vi "DoInit.vi"(8 "error in (no error)":errorcluster, 11 "Snake in":refnum<class "SnakeGame.lvclass">) -> (0 "error out":errorcluster, 3 "Snake out":refnum<class "SnakeGame.lvclass">)   [LabVIEW 2019, in "RT_Game.lvlib" / "SnakeGame.lvclass"]
uses:
  SnakeGame.lvclass
  C:/Users/FreshBob/Dropbox/VIs/myRIO_GameConsole/RT/RT_Game/Game/Game.lvclass
  SnakeData.ctl
  Direction.ctl
  Game/Coordinate.ctl
  CoordinateData.ctl
  RT_Sprite/RT_Sprite.lvclass
  C:/Users/FreshBob/Dropbox/VIs/myRIO_GameConsole/RT/RT_Game/GameObject/GameObject.lvclass
  PongSwitch/SnakeSwitch.lvclass
  Snake/Snake.lvclass
  SnakeGame.lvclass/SnakeGame.ctl
  GameObject/GameObject.lvclass/GameObject.ctl
  PongSwitch/SnakeSwitch.lvclass/SnakeSwitch.ctl
  Snake/Snake.lvclass/Snake.ctl
  Game/Game.lvclass/Game.ctl
  Snake/Write Position (Tiles).vi
  Snake/Write Direction.vi
  Snake/Write ScorePosition.vi
  Snake/Write Color.vi
  Snake/Write Length.vi
  GameObject/Write name.vi
  PongSwitch/Write Static.vi
  GameObject/Write IsActive.vi
  PongSwitch/Write DisabledTime.vi
  PongSwitch/Write EnabledTime.vi
  PongSwitch/Write randomness.vi
  GameObject/Write Collides_.vi
  Snake/Write Dead_.vi
  GameObject/Read position.vi
  Game/Write Sprites.vi
  Game/Game.lvclass
  GameObject/GameObject.lvclass
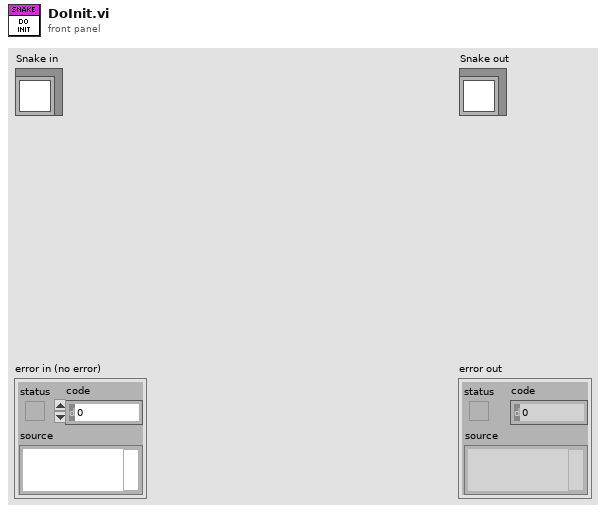
[diagram p1: front panel]
types:
  T1 = typedef "RT_Game.lvlib/Game.lvclass/Coordinate.ctl" = cluster{"x":dbl, "y":dbl}
  T2 = typedef "RT_Game.lvlib/SnakeGame.lvclass/Direction.ctl" = enum16{"Up", "Left", "Down", "Right"}
  T3 = typedef "RT_Game.lvlib/SnakeGame.lvclass/SnakeData.ctl" = cluster{"Length":i16, "Direction":T2, "Position":T1, "Coordinates":T4[], "ScorePosition":T1, "Dead?":bool, "Color":fxp<+,3,3>, "LastDirection":T2}
  T4 = typedef "RT_Game.lvlib/SnakeGame.lvclass/CoordinateData.ctl" = cluster{"Coordinate":T1, "TileCode":u16}
  T5 = cluster{"GameObject out":refnum<class "RT_Sprite.lvclass">, "GameObject out":refnum<class "RT_Sprite.lvclass">, "GameObject out":refnum<class "RT_Sprite.lvclass">}
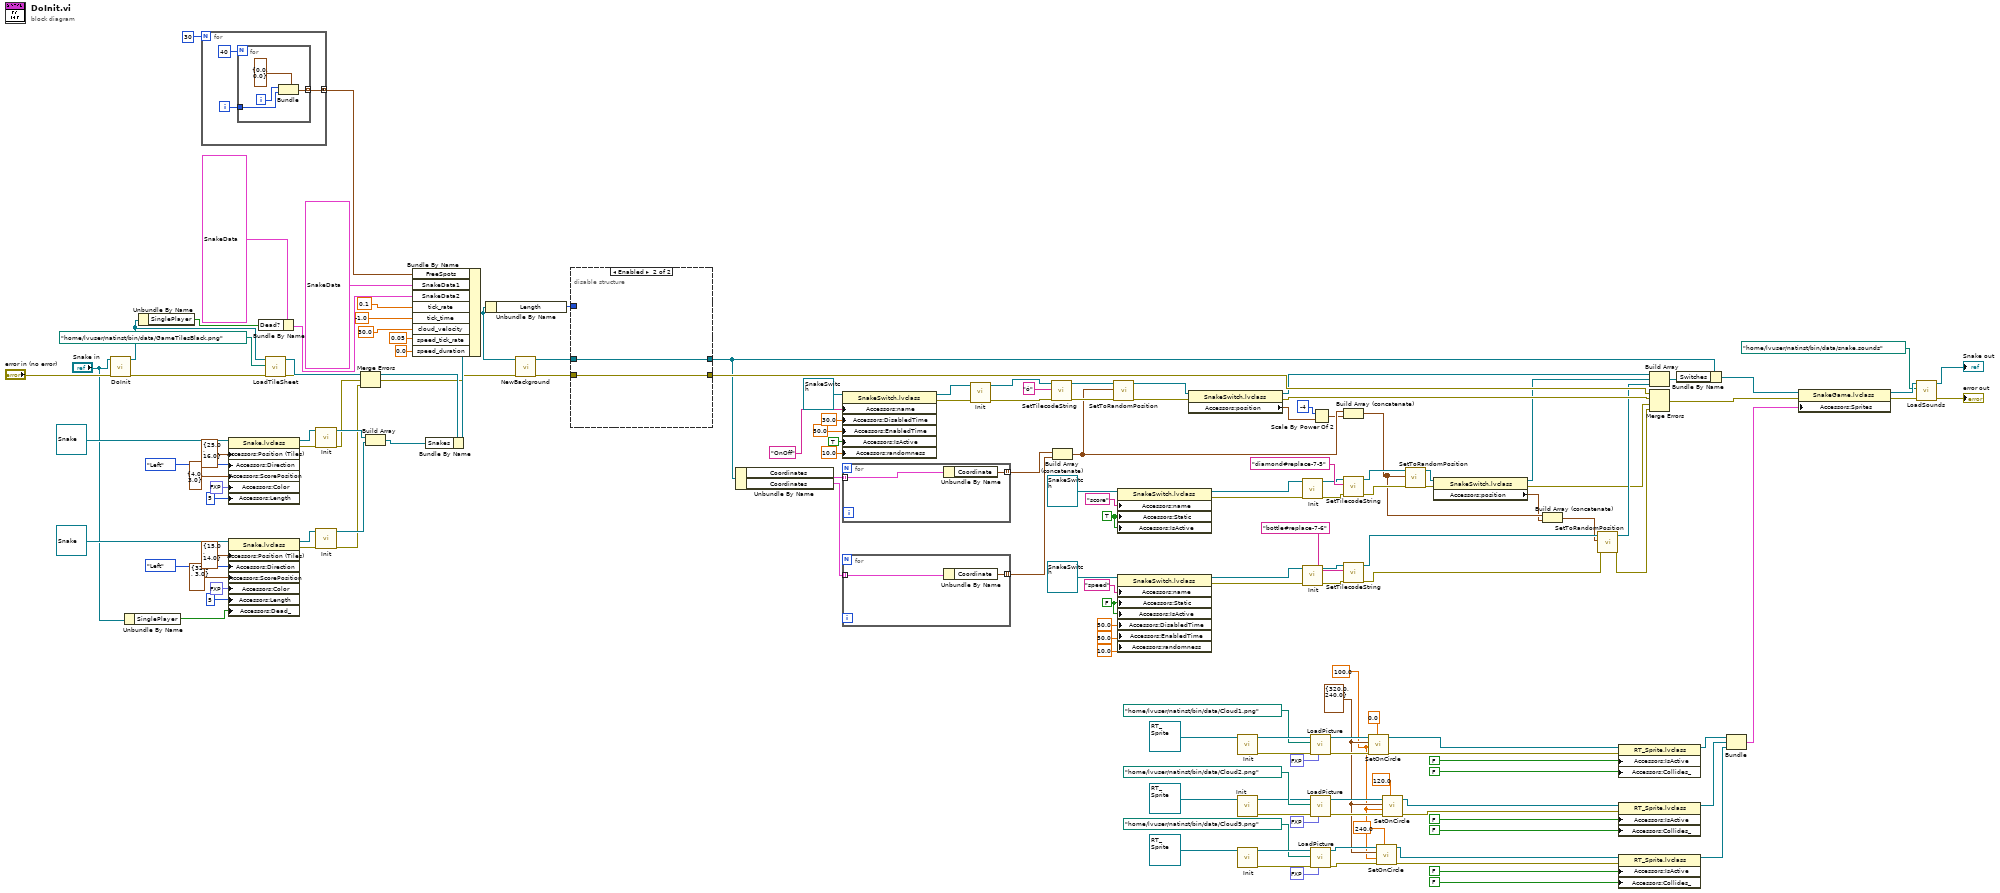
[diagram p0: block diagram]
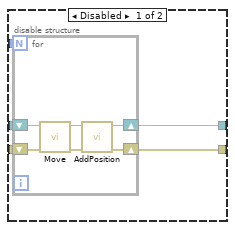
[diagram p2: hidden frame]
diagram:
  w52 = FALSE ("Static")
  w34 = TRUE ("Static")
  w65 = 100.0 ("Radius")
  w66 = T1 {"x"=320.0, "y"=240.0} ("Center")
  n1 = call-parent "DoInit.vi"("error in (no error)"="error in (no error)", "Game in"="Snake in") -> ("error out"=w153:errorcluster, "Game out"=w58:refnum<class "SnakeGame.lvclass">)  [unwired: 8 in]
  n2 = Unbundle By Name("Snake in") -> ("SinglePlayer"=w1:bool)
  n3 = Unbundle By Name(w58) -> ("SinglePlayer"=w146:bool)
  n4 = for {
    N: 30 -> [_]
    tunnel: [w156] -> w28 mode=concatenating
    i -> [w157]
    n5 = for {
      N: 40 -> [_]
      tunnel: w157 -> [w160]
      tunnel: [w159] -> w156 mode=indexing
      i -> [w161]
      n6 = Bundle(cluster=T1 {"x"=0.0, "y"=0.0} ("Coordinate"), "x"=w161, "y"=w160) -> (w159:T1)
    }
  }
  n7 = property class="Snake.lvclass"(reference=refnum<class "Snake.lvclass"> refnum ("RT_Game.lvlib:Snake.lvclass"), "Accessors:Position (Tiles)"=T1 {"x"=25.0, "y"=16.0} ("Position (Tiles)"), "Accessors:Direction"=Direction."Left" ("Direction"), "Accessors:ScorePosition"=T1 {"x"=4.0, "y"=3.0} ("ScorePosition"), "Accessors:Color"=fxp<+,3,3> 1.0 ("Color"), "Accessors:Length"=i16 5 ("Length")) -> (reference out=w24:refnum<class "Snake.lvclass">, error out=w23:errorcluster)  [unwired: 1 in]
  n8 = property class="Snake.lvclass"(reference=refnum<class "Snake.lvclass"> refnum ("RT_Game.lvlib:Snake.lvclass"), "Accessors:Position (Tiles)"=T1 {"x"=15.0, "y"=14.0} ("Position (Tiles)"), "Accessors:Direction"=Direction."Left" ("Direction"), "Accessors:ScorePosition"=T1 {"x"=32.0, "y"=3.0} ("ScorePosition"), "Accessors:Color"=fxp<+,3,3> 2.0 ("Color"), "Accessors:Length"=i16 5 ("Length"), "Accessors:Dead_"=w1) -> (reference out=w11:refnum<class "Snake.lvclass">, error out=w12:errorcluster)  [unwired: 1 in]
  n9 = Bundle By Name(cluster=T3 {"Length"=5, "Direction"=enum."Right", "Position"={"x"=15.0, "y"=14.0}, "Coordinates"=[], "ScorePosition"={"x"=32.0, "y"=3.0}, "Dead?"=FALSE, "Color"=2.0, "LastDirection"=enum."Up"} ("SnakeData1"), "Dead?"=w146) -> (w147:T3)
  n10 = call "LoadTileSheet.vi"("error in (no error)"=w153, "Tile Path"=path "/home/lvuser/natinst/bin/data/GameTilesBlack.png", "Game in"=w58) -> ("error out"=w116:errorcluster, "Game out"=w117:refnum<class "SnakeGame.lvclass">)  [unwired: 7 in]
  n11 = call-dynamic "Init.vi"("error in (no error)"=w23, "Snake in"=w24) -> ("error out"=w5:errorcluster, "Snake out"=w8:refnum<class "Snake.lvclass">)  [unwired: 8 in]
  n12 = call-dynamic "Init.vi"("error in (no error)"=w12, "Snake in"=w11) -> ("error out"=w4:errorcluster, "Snake out"=w7:refnum<class "Snake.lvclass">)  [unwired: 8 in]
  n13 = Merge Errors(w116, w5, w4) -> (w6:errorcluster)
  n14 = Build Array(w8, w7) -> (w3:refnum<class "Snake.lvclass">[])
  n15 = Bundle By Name(cluster=w117, "Snakes"=w3) -> (w9:refnum<class "SnakeGame.lvclass">)
  n16 = Bundle By Name(cluster=w9, "FreeSpots"=w28, "SnakeData1"=T3 {"Length"=5, "Direction"=enum."Left", "Position"={"x"=25.0, "y"=16.0}, "Coordinates"=[], "ScorePosition"={"x"=4.0, "y"=3.0}, "Dead?"=FALSE, "Color"=1.0, "LastDirection"=enum."Up"}, "SnakeData2"=w147, "tick_rate"=0.1, "tick_time"=-1.0, "cloud_velocity"=30.0, "speed_tick_rate"=0.05, "speed_duration"=0.0) -> (w150:refnum<class "SnakeGame.lvclass">)
  n17 = Unbundle By Name(w150) -> ("Length"=w154:i16)
  n18 = call "NewBackground.vi"("error in (no error)"=w6, "Snake in"=w150) -> ("error out"=w151:errorcluster, "Snake out"=w152:refnum<class "SnakeGame.lvclass">)  [unwired: 8 in]
  n19 = disable-structure shown="Enabled" {
    disable-tunnel: w154 -> [w167 _]
    disable-tunnel: w152 -> [w166 w175]
    disable-tunnel: w151 -> [w165 w174]
    disable-tunnel: [w164 w174] -> w114
    disable-tunnel: [w163 w175] -> w110
    frame Disabled {
      n20 = for {
        N: w167 -> [_]
        shift-right: [w168] -> w163
        shift-left: w166 -> [w173]
        shift-right: [w170] -> w164
        shift-left: w165 -> [w172]
        n21 = call "Move.vi"("error in (no error)"=w172, "Snake in"=w173) -> ("error out"=w171:errorcluster, "Snake out"=w169:refnum<class "SnakeGame.lvclass">)  [unwired: 8 in]
        n22 = call "AddPosition.vi"("error in (no error)"=w171, "Snake in"=w169) -> ("error out"=w170:errorcluster, "Snake out"=w168:refnum<class "SnakeGame.lvclass">)  [unwired: 8 in]
      }
    }
    frame Enabled {
    }
  }
  n23 = Unbundle By Name(w110) -> ("Coordinates"=w109:T4[], "Coordinates"=w107:T4[])
  n24 = property class="SnakeSwitch.lvclass"(reference=refnum<class "SnakeSwitch.lvclass"> refnum ("RT_Game.lvlib:SnakeSwitch.lvclass"), "Accessors:name"="OnOff" ("name"), "Accessors:DisabledTime"=30.0 ("DisabledTime"), "Accessors:EnabledTime"=50.0 ("EnabledTime"), "Accessors:IsActive"=TRUE ("IsActive"), "Accessors:randomness"=10.0 ("randomness")) -> (reference out=w124:refnum<class "SnakeSwitch.lvclass">, error out=w120:errorcluster)  [unwired: 1 in]
  n25 = for {
    tunnel: w109 -> [w177] mode=indexing
    tunnel: [w176] -> w108 mode=indexing
    n26 = Unbundle By Name(w177) -> ("Coordinate"=w176:T1)
  }
  n27 = for {
    tunnel: w107 -> [w179] mode=indexing
    tunnel: [w178] -> w104 mode=indexing
    n28 = Unbundle By Name(w179) -> ("Coordinate"=w178:T1)
  }
  n29 = call-dynamic "Init.vi"("error in (no error)"=w120, "PongSwitch in"=w124) -> ("error out"=w133:errorcluster, "PongSwitch out"=w132:refnum<class "SnakeSwitch.lvclass">)  [unwired: 8 in]
  n30 = call "SetTilecodeString.vi"("error in (no error)"=w133, "TileCode"="ó", "PongSwitch in"=w132) -> ("error out"=w106:errorcluster, "PongSwitch out"=w105:refnum<class "SnakeSwitch.lvclass">)  [unwired: 7 in]
  n31 = Build Array (concatenate)(w108, w104) -> (w100:T1[])
  n32 = call "SetToRandomPosition.vi"("error in (no error)"=w106, "BlockedSpots"=w100, "SnakeSwitch in"=w105) -> ("error out"=w118:errorcluster, "SnakeSwitch out"=w102:refnum<class "SnakeSwitch.lvclass">)  [unwired: 7 in]
  n33 = property class="SnakeSwitch.lvclass"(reference=refnum<class "SnakeSwitch.lvclass"> refnum ("RT_Game.lvlib:SnakeSwitch.lvclass"), "Accessors:name"="score" ("name"), "Accessors:Static"=w34, "Accessors:IsActive"=w34) -> (reference out=w122:refnum<class "SnakeSwitch.lvclass">, error out=w119:errorcluster)  [unwired: 1 in]
  n34 = property class="SnakeSwitch.lvclass"(reference=refnum<class "SnakeSwitch.lvclass"> refnum ("RT_Game.lvlib:SnakeSwitch.lvclass"), "Accessors:name"="speed" ("name"), "Accessors:Static"=w52, "Accessors:IsActive"=w52, "Accessors:DisabledTime"=50.0 ("DisabledTime"), "Accessors:EnabledTime"=50.0 ("EnabledTime"), "Accessors:randomness"=10.0 ("randomness")) -> (reference out=w48:refnum<class "SnakeSwitch.lvclass">, error out=w50:errorcluster)  [unwired: 1 in]
  n35 = property class="SnakeSwitch.lvclass"(reference=w102, error in=w118) -> (reference out=w101:refnum<class "SnakeSwitch.lvclass">, error out=w103:errorcluster, "Accessors:position"=w99:T1)
  n36 = call-dynamic "Init.vi"("RT_Sprite in"=refnum<class "RT_Sprite.lvclass"> refnum ("RT_Game.lvlib:RT_Sprite.lvclass")) -> ("error out"=w140:errorcluster, "RT_Sprite out"=w141:refnum<class "RT_Sprite.lvclass">)  [unwired: 9 in]
  n37 = call-dynamic "Init.vi"("RT_Sprite in"=refnum<class "RT_Sprite.lvclass"> refnum ("RT_Game.lvlib:RT_Sprite.lvclass")) -> ("error out"=w93:errorcluster, "RT_Sprite out"=w92:refnum<class "RT_Sprite.lvclass">)  [unwired: 9 in]
  n38 = call-dynamic "Init.vi"("RT_Sprite in"=refnum<class "RT_Sprite.lvclass"> refnum ("RT_Game.lvlib:RT_Sprite.lvclass")) -> ("error out"=w88:errorcluster, "RT_Sprite out"=w89:refnum<class "RT_Sprite.lvclass">)  [unwired: 9 in]
  n39 = call-dynamic "Init.vi"("error in (no error)"=w119, "PongSwitch in"=w122) -> ("error out"=w128:errorcluster, "PongSwitch out"=w129:refnum<class "SnakeSwitch.lvclass">)  [unwired: 8 in]
  n40 = call-dynamic "Init.vi"("error in (no error)"=w50, "PongSwitch in"=w48) -> ("error out"=w45:errorcluster, "PongSwitch out"=w44:refnum<class "SnakeSwitch.lvclass">)  [unwired: 8 in]
  n41 = call "LoadPicture.vi"("Transparent Color"=fxp<+,3,3> 0.0, "error in (no error)"=w140, "Picture Path"=path "/home/lvuser/natinst/bin/data/Cloud1.png" ("Tile Path"), "RT_Sprite in"=w141) -> ("error out"=w137:errorcluster, "RT_Sprite out"=w82:refnum<class "RT_Sprite.lvclass">)  [unwired: 6 in]
  n42 = call "LoadPicture.vi"("Transparent Color"=fxp<+,3,3> 0.0, "error in (no error)"=w93, "Picture Path"=path "/home/lvuser/natinst/bin/data/Cloud2.png" ("Tile Path"), "RT_Sprite in"=w92) -> ("error out"=w81:errorcluster, "RT_Sprite out"=w95:refnum<class "RT_Sprite.lvclass">)  [unwired: 6 in]
  n43 = call "LoadPicture.vi"("Transparent Color"=fxp<+,3,3> 0.0, "error in (no error)"=w88, "Picture Path"=path "/home/lvuser/natinst/bin/data/Cloud9.png" ("Tile Path"), "RT_Sprite in"=w89) -> ("error out"=w86:errorcluster, "RT_Sprite out"=w68:refnum<class "RT_Sprite.lvclass">)  [unwired: 6 in]
  n44 = Scale By Power Of 2(n=i16 -4, x=w99) -> (x*2^n=w97:T1)
  n45 = Build Array (concatenate)(w100, w97) -> (w37:T1[])
  n46 = call "SetTilecodeString.vi"("error in (no error)"=w128, "TileCode"="diamond#replace-7-5", "PongSwitch in"=w129) -> ("error out"=w126:errorcluster, "PongSwitch out"=w111:refnum<class "SnakeSwitch.lvclass">)  [unwired: 7 in]
  n47 = call "SetTilecodeString.vi"("error in (no error)"=w45, "TileCode"="bottle#replace-7-6", "PongSwitch in"=w44) -> ("error out"=w47:errorcluster, "PongSwitch out"=w51:refnum<class "SnakeSwitch.lvclass">)  [unwired: 7 in]
  n48 = call "SetOnCircle.vi"("angle (deg)"=0.0, "error in (no error)"=w137, "Radius"=w65, "Center"=w66, "GameObject in"=w82) -> ("error out"=w72:errorcluster, "GameObject out"=w73:refnum<class "RT_Sprite.lvclass">)  [unwired: 5 in]
  n49 = call "SetOnCircle.vi"("angle (deg)"=240.0, "error in (no error)"=w86, "Radius"=w65, "Center"=w66, "GameObject in"=w68) -> ("error out"=w69:errorcluster, "GameObject out"=w67:refnum<class "RT_Sprite.lvclass">)  [unwired: 5 in]
  n50 = call "SetOnCircle.vi"("angle (deg)"=120.0, "error in (no error)"=w81, "Radius"=w65, "Center"=w66, "GameObject in"=w95) -> ("error out"=w70:errorcluster, "GameObject out"=w71:refnum<class "RT_Sprite.lvclass">)  [unwired: 5 in]
  n51 = call "SetToRandomPosition.vi"("error in (no error)"=w126, "BlockedSpots"=w37, "SnakeSwitch in"=w111) -> ("error out"=w112:errorcluster, "SnakeSwitch out"=w39:refnum<class "SnakeSwitch.lvclass">)  [unwired: 7 in]
  n52 = property class="SnakeSwitch.lvclass"(reference=w39, error in=w112) -> (reference out=w38:refnum<class "SnakeSwitch.lvclass">, error out=w40:errorcluster, "Accessors:position"=w36:T1)
  n53 = Build Array (concatenate)(w37, w36) -> (w35:T1[])
  n54 = call "SetToRandomPosition.vi"("error in (no error)"=w47, "BlockedSpots"=w35, "SnakeSwitch in"=w51) -> ("error out"=w42:errorcluster, "SnakeSwitch out"=w41:refnum<class "SnakeSwitch.lvclass">)  [unwired: 7 in]
  n55 = property class="RT_Sprite.lvclass"(reference=w73, error in=w72, "Accessors:IsActive"=FALSE ("IsActive"), "Accessors:Collides_"=FALSE ("Collides_")) -> (reference out=w76:refnum<class "RT_Sprite.lvclass">)  [unwired: 1 out]
  n56 = property class="RT_Sprite.lvclass"(reference=w71, error in=w70, "Accessors:IsActive"=FALSE ("IsActive"), "Accessors:Collides_"=FALSE ("Collides_")) -> (reference out=w75:refnum<class "RT_Sprite.lvclass">)  [unwired: 1 out]
  n57 = property class="RT_Sprite.lvclass"(reference=w67, error in=w69, "Accessors:IsActive"=FALSE ("IsActive"), "Accessors:Collides_"=FALSE ("Collides_")) -> (reference out=w74:refnum<class "RT_Sprite.lvclass">)  [unwired: 1 out]
  n58 = Build Array(w101, w38, w41) -> (w125:refnum<class "SnakeSwitch.lvclass">[])
  n59 = Merge Errors(w114, w103, w40, w42) -> (w113:errorcluster)
  n60 = Bundle By Name(cluster=w110, "Switches"=w125) -> (w115:refnum<class "SnakeGame.lvclass">)
  n61 = Bundle("GameObject out"=w76, "GameObject out"=w75, "GameObject out"=w74) -> (w138:T5)  [unwired: 1 in]
  n62 = property class="SnakeGame.lvclass"(reference=w115, error in=w113, "Accessors:Sprites"=w138) -> (reference out=w60:refnum<class "SnakeGame.lvclass">, error out=w143:errorcluster)
  n63 = call "LoadSounds.vi"("error in (no error)"=w143, "Path"=path "/home/lvuser/natinst/bin/data/snake.sounds", "Game in"=w60) -> ("error out"=→"error out":errorcluster, "Game out"=→"Snake out":refnum<class "SnakeGame.lvclass">)  [unwired: 7 in]
